vi "UpdateTime.vi"(8 "error in (no error)":errorcluster, 10 "SnakeGame in":refnum<class "SnakeGame.lvclass">, 11 "SnakeSwitch in":refnum<class "SnakeSwitch.lvclass">) -> (0 "error out":errorcluster, 2 "SnakeGame out":refnum<class "SnakeGame.lvclass">, 3 "SnakeSwitch out":refnum<class "SnakeSwitch.lvclass">)   [LabVIEW 2019, in "RT_Game.lvlib" / "SnakeSwitch.lvclass"]
uses:
  SnakeSwitch.lvclass
  C:/Users/FreshBob/Dropbox/VIs/myRIO_GameConsole/RT/RT_Game/GameObject/GameObject.lvclass
  SnakeGame/SnakeGame.lvclass
  SnakeSwitch.lvclass/SnakeSwitch.ctl
  GameObject/GameObject.lvclass/GameObject.ctl
  GameObject/Write IsActive.vi
  GameObject/Read IsActive.vi
  Globals.vi
  RT_Game.lvlib
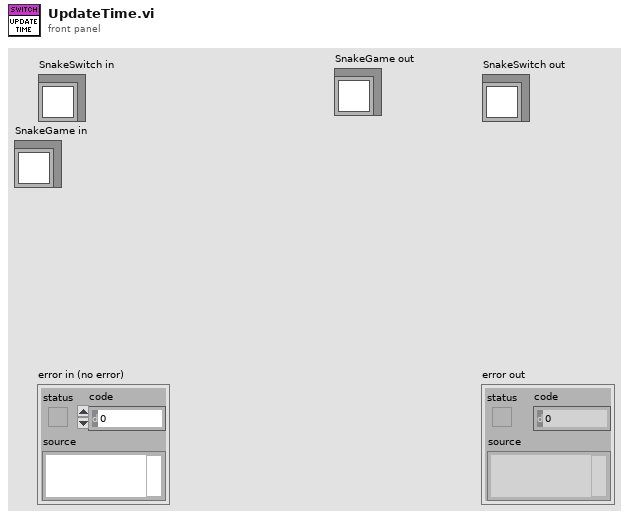
[diagram p1: front panel]
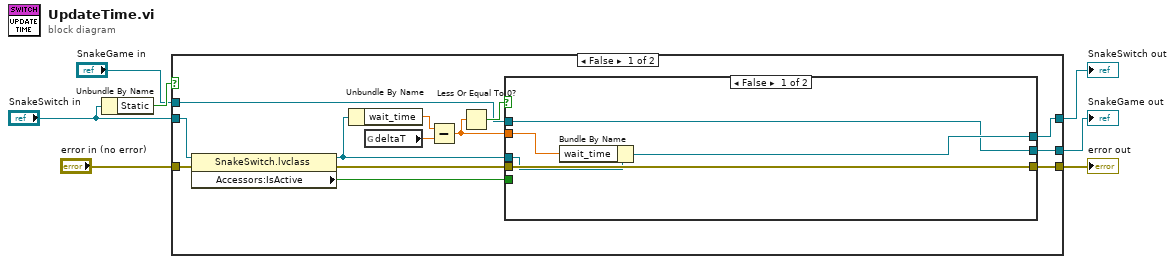
[diagram p0: block diagram]
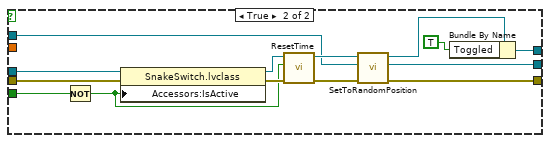
[diagram p2: hidden frame]
diagram:
  n1 = Unbundle By Name("SnakeSwitch in") -> ("Static"=w5:bool)
  n2 = case shown="False" w5 {
    tunnel: "error in (no error)" -> [w20 w41]
    tunnel: "SnakeSwitch in" -> [w17 w42]
    tunnel: [w14 w42] -> w6
    tunnel: [w11 w41] -> w4
    tunnel: [w9 w40] -> w2
    tunnel: "SnakeGame in" -> [w8 w40]
    frame False {
      n3 = property class="SnakeSwitch.lvclass"(reference=w17, error in=w20) -> (reference out=w15:refnum<class "SnakeSwitch.lvclass">, error out=w18:errorcluster, "Accessors:IsActive"=w16:bool)
      n4 = Unbundle By Name(w15) -> ("wait_time"=w19:dbl)
      n5 = global read "Globals.vi" "deltaT"() -> (w10:dbl)
      n6 = Subtract(x=w19, y=w10) -> (x-y=w13:dbl)
      n7 = Less Or Equal To 0?(x=w13) -> (x <= 0?=w12:bool)
      n8 = case shown="False" w12 {
        tunnel: w13 -> [w22 _]
        tunnel: w18 -> [w25 w39]
        tunnel: [w25 w31] -> w11
        tunnel: w16 -> [_ w37]
        tunnel: w15 -> [w24 w36]
        tunnel: [w23 w35] -> w14
        tunnel: [w21 w27] -> w9
        tunnel: w8 -> [w21 w26]
        frame False {
          n9 = Bundle By Name(cluster=w24, "wait_time"=w22) -> (w23:refnum<class "SnakeSwitch.lvclass">)
        }
        frame True {
          n10 = Not(x=w37) -> (.not. x?=w28:bool)
          n11 = property class="SnakeSwitch.lvclass"(reference=w36, error in=w39, "Accessors:IsActive"=w28) -> (reference out=w32:refnum<class "SnakeSwitch.lvclass">, error out=w38:errorcluster)
          n12 = call "ResetTime.vi"("error in (no error)"=w38, "enabled"=w28, "SnakeSwitch in"=w32) -> ("error out"=w33:errorcluster, "SnakeSwitch out"=w30:refnum<class "SnakeSwitch.lvclass">)  [unwired: 7 in]
          n13 = call "SetToRandomPosition.vi"("error in (no error)"=w33, "SnakeGame in"=w26, "SnakeSwitch in"=w30) -> ("error out"=w31:errorcluster, "SnakeGame out"=w27:refnum<class "SnakeGame.lvclass">, "SnakeSwitch out"=w29:refnum<class "SnakeSwitch.lvclass">)  [unwired: 6 in]
          n14 = Bundle By Name(cluster=w29, "Toggled"=TRUE) -> (w35:refnum<class "SnakeSwitch.lvclass">)
        }
      }
    }
    frame True {
    }
  }
  "SnakeSwitch out" <- w6
  "error out" <- w4
  "SnakeGame out" <- w2
